vi "Run VI from Path.vi"(8 "error in (no error)":errorcluster, 11 "vi path":path) -> (0 "error out":errorcluster, 3 "type specifier VI Refnum (for type only)":refnum<vi>)   [LabVIEW 2017]
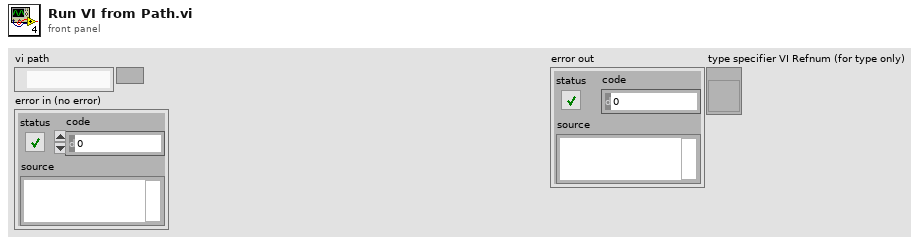
[diagram p1: front panel]
types:
  T1 = enum32{"Bad", "Idle", "Run top level", "Running"}
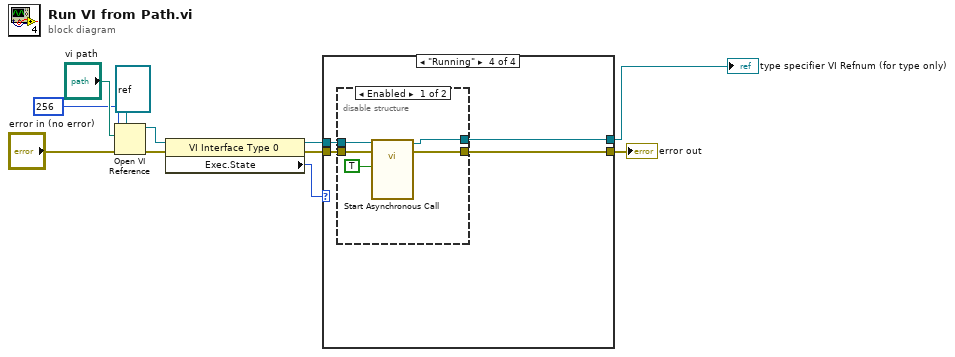
[diagram p0: block diagram]
diagram:
  n1 = Open VI Reference(type specifier VI Refnum (for type only)=refnum<vi> refnum, vi path="vi path", options=256, error in (no error)="error in (no error)") -> (vi reference=w6:refnum<vi>, error out=w8:errorcluster)  [unwired: 2 in]
  n2 = property class="VI Interface Type 0"(reference=w6, error in=w8) -> (reference out=w4:refnum<vi>, error out=w7:errorcluster, "Exec.State"=w5:T1)
  n3 = case shown="\"Running\"" w5 {
    tunnel: w7 -> [w13 w15 w17 w21]
    tunnel: w4 -> [w12 w14 w16 w20]
    tunnel: [w13 w15 w17 w19] -> w3
    tunnel: [w12 w14 w16 w18] -> w1
    frame "Bad", Default {
    }
    frame "Idle" {
    }
    frame "Run top level" {
    }
    frame "Running" {
      n4 = disable-structure shown="Enabled" {
        disable-tunnel: w21 -> [w25 w28]
        disable-tunnel: w20 -> [w24 w27]
        disable-tunnel: [w23 w28] -> w19
        disable-tunnel: [w22 w27] -> w18
        frame Enabled {
          n5 = call-by-ref "Start Asynchronous Call"(reference=w24, error in=w25, "Remote?"=TRUE) -> (reference out=w22:refnum<vi>, error out=w23:errorcluster)  [unwired: 11 in]
        }
        frame Disabled {
        }
      }
    }
  }
  "error out" <- w3
  "type specifier VI Refnum (for type only)" <- w1
